vi "Conf Gemeral.vi"(8 "error in (no error)":errorcluster, 11 "Conf. Gral.":T1) -> (0 "error out":errorcluster, 3 "Conf. Gral. Out":T1)   [LabVIEW 2014, in "MathLoop.lvlib"]
uses:
  MathLoop.lvlib
  TypeDefs/Conf. Gral.ctl
panel:
  in  "Cant. Dientes x pieza:":i32
  in  "Nro. de Dientes:":i32
  in  "Acept":bool
  in  "Cancelar":bool
  in  "Armonicos:":i32
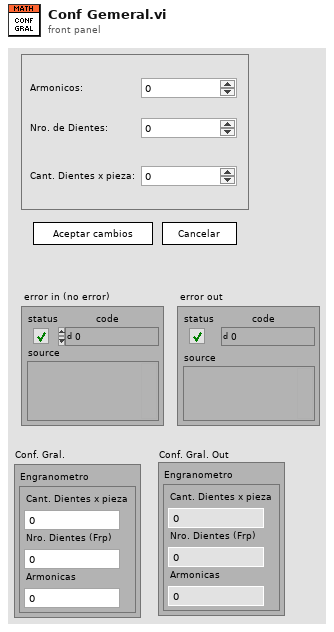
[diagram p1: front panel]
types:
  T1 = typedef "MathLoop.lvlib/Conf. Gral.ctl" = cluster{"Engranometro":cluster{"Cant. Dientes x pieza":i32, "Nro. Dientes (Frp)":i32, "Armonicas":i32}}
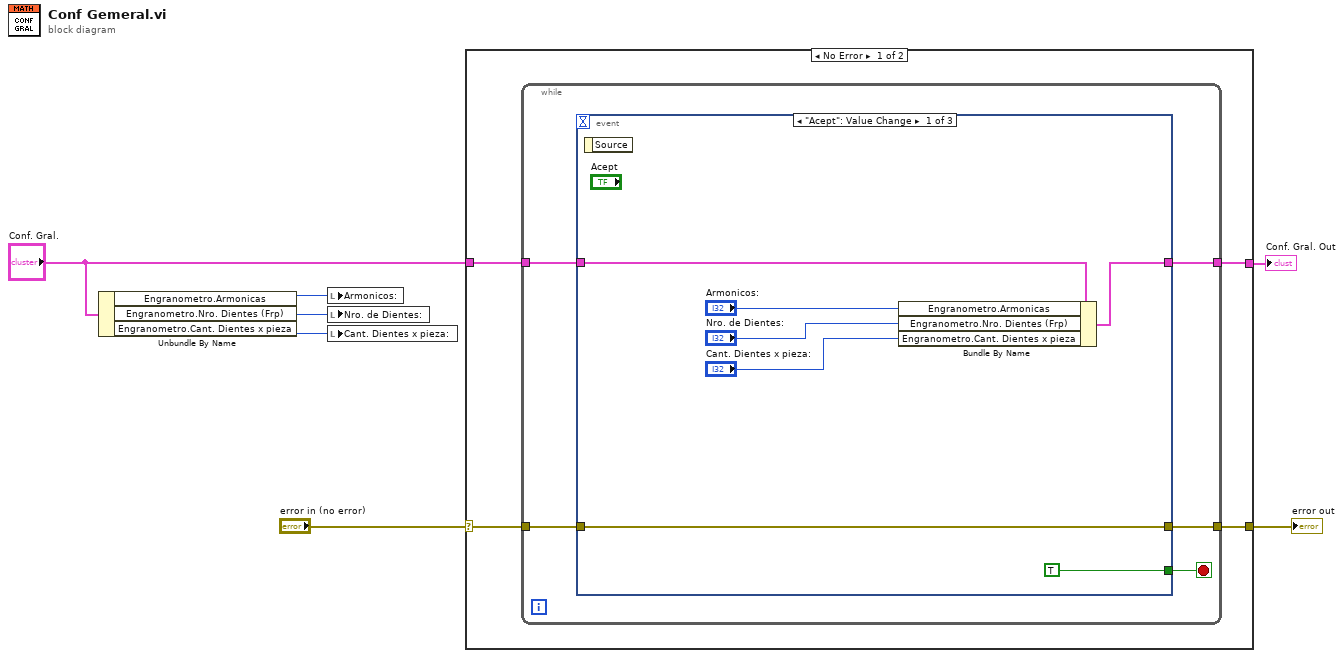
[diagram p0: block diagram]
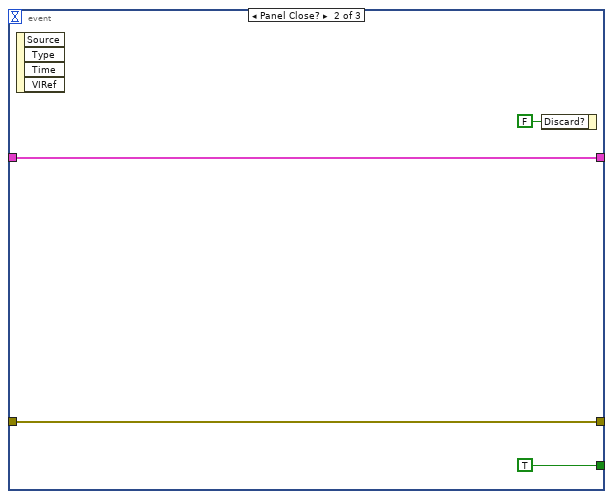
[diagram p2: hidden frame]
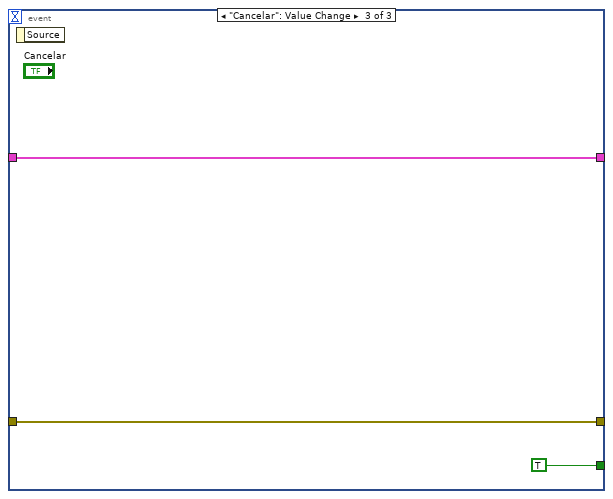
[diagram p3: hidden frame]
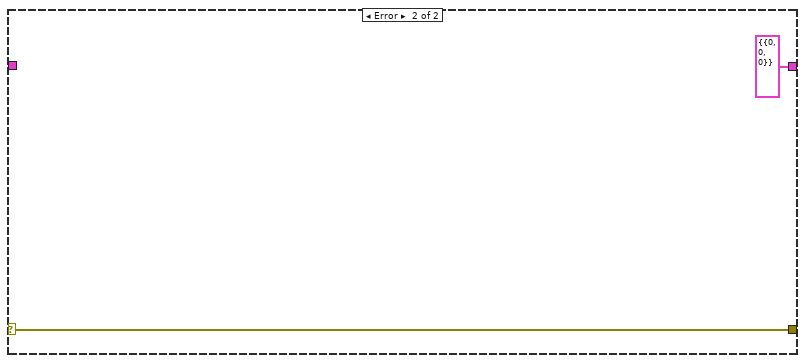
[diagram p4: hidden frame]
diagram:
  n1 = Unbundle By Name("Conf. Gral.") -> ("Engranometro.Armonicas"=w4:i32, "Engranometro.Nro. Dientes (Frp)"=w3:i32, "Engranometro.Cant. Dientes x pieza"=w2:i32)
  n2 = local write "Armonicos:"(w4) -> ()
  n3 = local write "Nro. de Dientes:"(w3) -> ()
  n4 = local write "Cant. Dientes x pieza:"(w2) -> ()
  n5 = case shown="No Error" "error in (no error)" {
    selector: "error in (no error)" -> [w10 w32]
    tunnel: [w11 w32] -> w6
    tunnel: "Conf. Gral." -> [w9 _]
    tunnel: [w8 T1 {"Engranometro"={"Cant. Dientes x pieza"=0, "Nro. Dientes (Frp)"=0, "Armonicas"=0}} ("Conf. Gral.")] -> w1
    frame No Error {
      n6 = while {
        tunnel: [w15] -> w11
        tunnel: w10 -> [w14]
        tunnel: w9 -> [w13]
        tunnel: [w12] -> w8
        stop <- w16 stop-if-true
        n7 = event shown="[0] \"Acept\": Value Change" {
          selector: _ -> [_ _ _]
          dyn-events: _ -> [_ _ _]
          timeout: _ -> [_ _ _]
          tunnel: [TRUE ("Discard?") TRUE ("Discard?") TRUE ("Discard?")] -> w16
          tunnel: [w22 w25 w29] -> w15
          tunnel: w14 -> [w22 w25 w29]
          tunnel: w13 -> [w21 w24 w28]
          tunnel: [w20 w24 w28] -> w12
          event "Acept": Value Change {
            n8 = event-data() -> ()  [unwired: 1 in, 1 out]
            n9 = Bundle By Name(cluster=w21, "Engranometro.Armonicas"="Armonicos:", "Engranometro.Nro. Dientes (Frp)"="Nro. de Dientes:", "Engranometro.Cant. Dientes x pieza"="Cant. Dientes x pieza:") -> (w20:T1)
          }
          event Panel Close? {
            n10 = event-data() -> ()  [unwired: 1 in, 4 out]
            n11 = event-data("Discard?"=FALSE) -> ()  [unwired: 1 in, 1 out]
          }
          event "Cancelar": Value Change {
            n12 = event-data() -> ()  [unwired: 1 in, 1 out]
          }
        }
      }
    }
    frame Error {
    }
  }
  "error out" <- w6
  "Conf. Gral. Out" <- w1
